vi "display_michelle_PKT_visjitter_stopadded_RandCont_PsuedoCO_TSLogFC2_lightdetection.vi"() -> ()   [LabVIEW 2019]
uses:
  <vilib>/Analysis/Matrix/Datatypes/RealMatrix.ctl
  <vilib>/Utility/file.llb/Write Delimited Spreadsheet (DBL).vi
  <vilib>/Analysis/Matrix/NI_Matrix.lvlib
panel:
  out "LastTimeOutTime":dbl
  out "lambda":dbl
  out "maxITI":dbl
  out "minITI":dbl
  out "goEXP":dbl
  out "meanITI":dbl
  out "Lag1":dbl
  out "TSLog":dbl[][](array[numeric])
  out "TSLog2":dbl[][](array[numeric])
  out "Initialtime":dbl
  out "Time Stamp":timestamp format="%<%H:%M:%S%4u>T"
  out "TSLog1":dbl[][](array[numeric])
  out "ArrayTemp3":T1
  out "StimID2":dbl
  out "Contrast":dbl
  out "TimeOutCounter":i32
  out "ElapsedTime_M":dbl
  out "Base_Contrast":dbl
  out "CurrentTrial":u32=1
  out "Jitter":dbl
  out "BaseITI":dbl
  out "VisStimDuration":dbl
  in  "Stop":bool
  out "Num trials":u32=204
  out "ISI Time":dbl
  out "Stim TS":dbl
  out "Output":dbl[][](array[numeric])
  out "Output frame":T1
  out "Array temp1":T1
  out "Elapsed Time":dbl
  out "Display":bool=TRUE
  out "Trial":u32=1
  out "reward":dbl[](array[numeric])
  out "stim_id":dbl[](array[numeric])
  out "stim_loaded":dbl
  out "Timings":dbl[](array[numeric])
  out "Stimuli Loaded?":bool
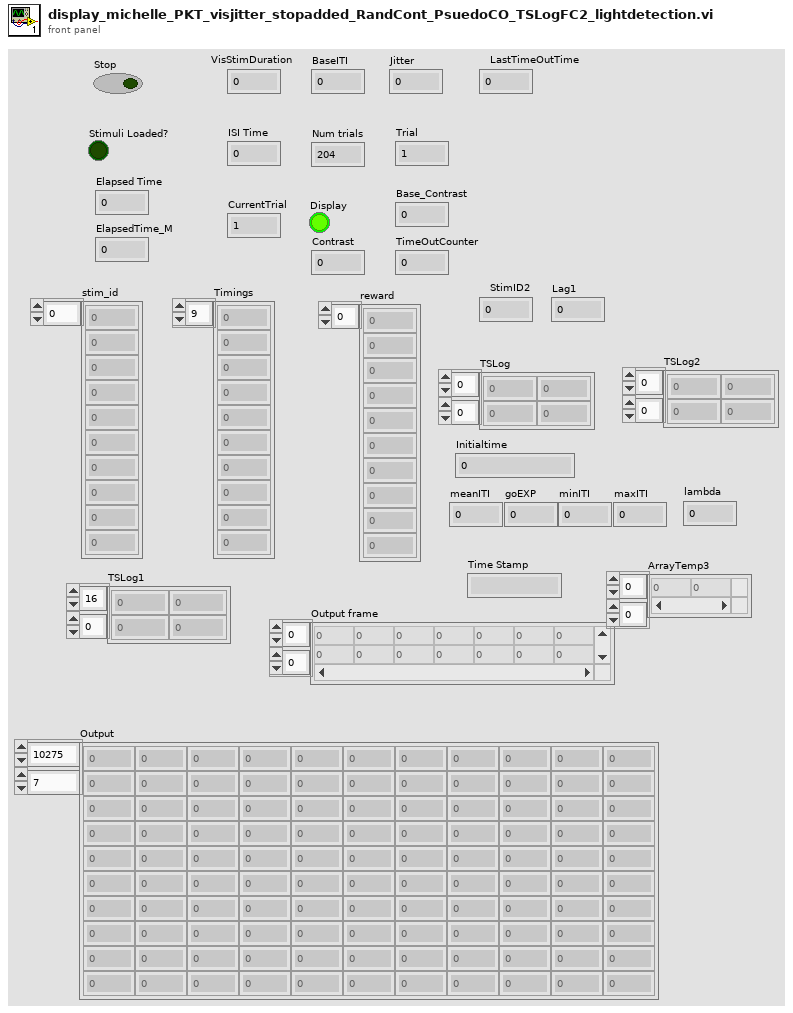
[diagram p1: front panel]
types:
  T1 = typedef "NI_Matrix.lvlib/RealMatrix.ctl" = dbl[][]
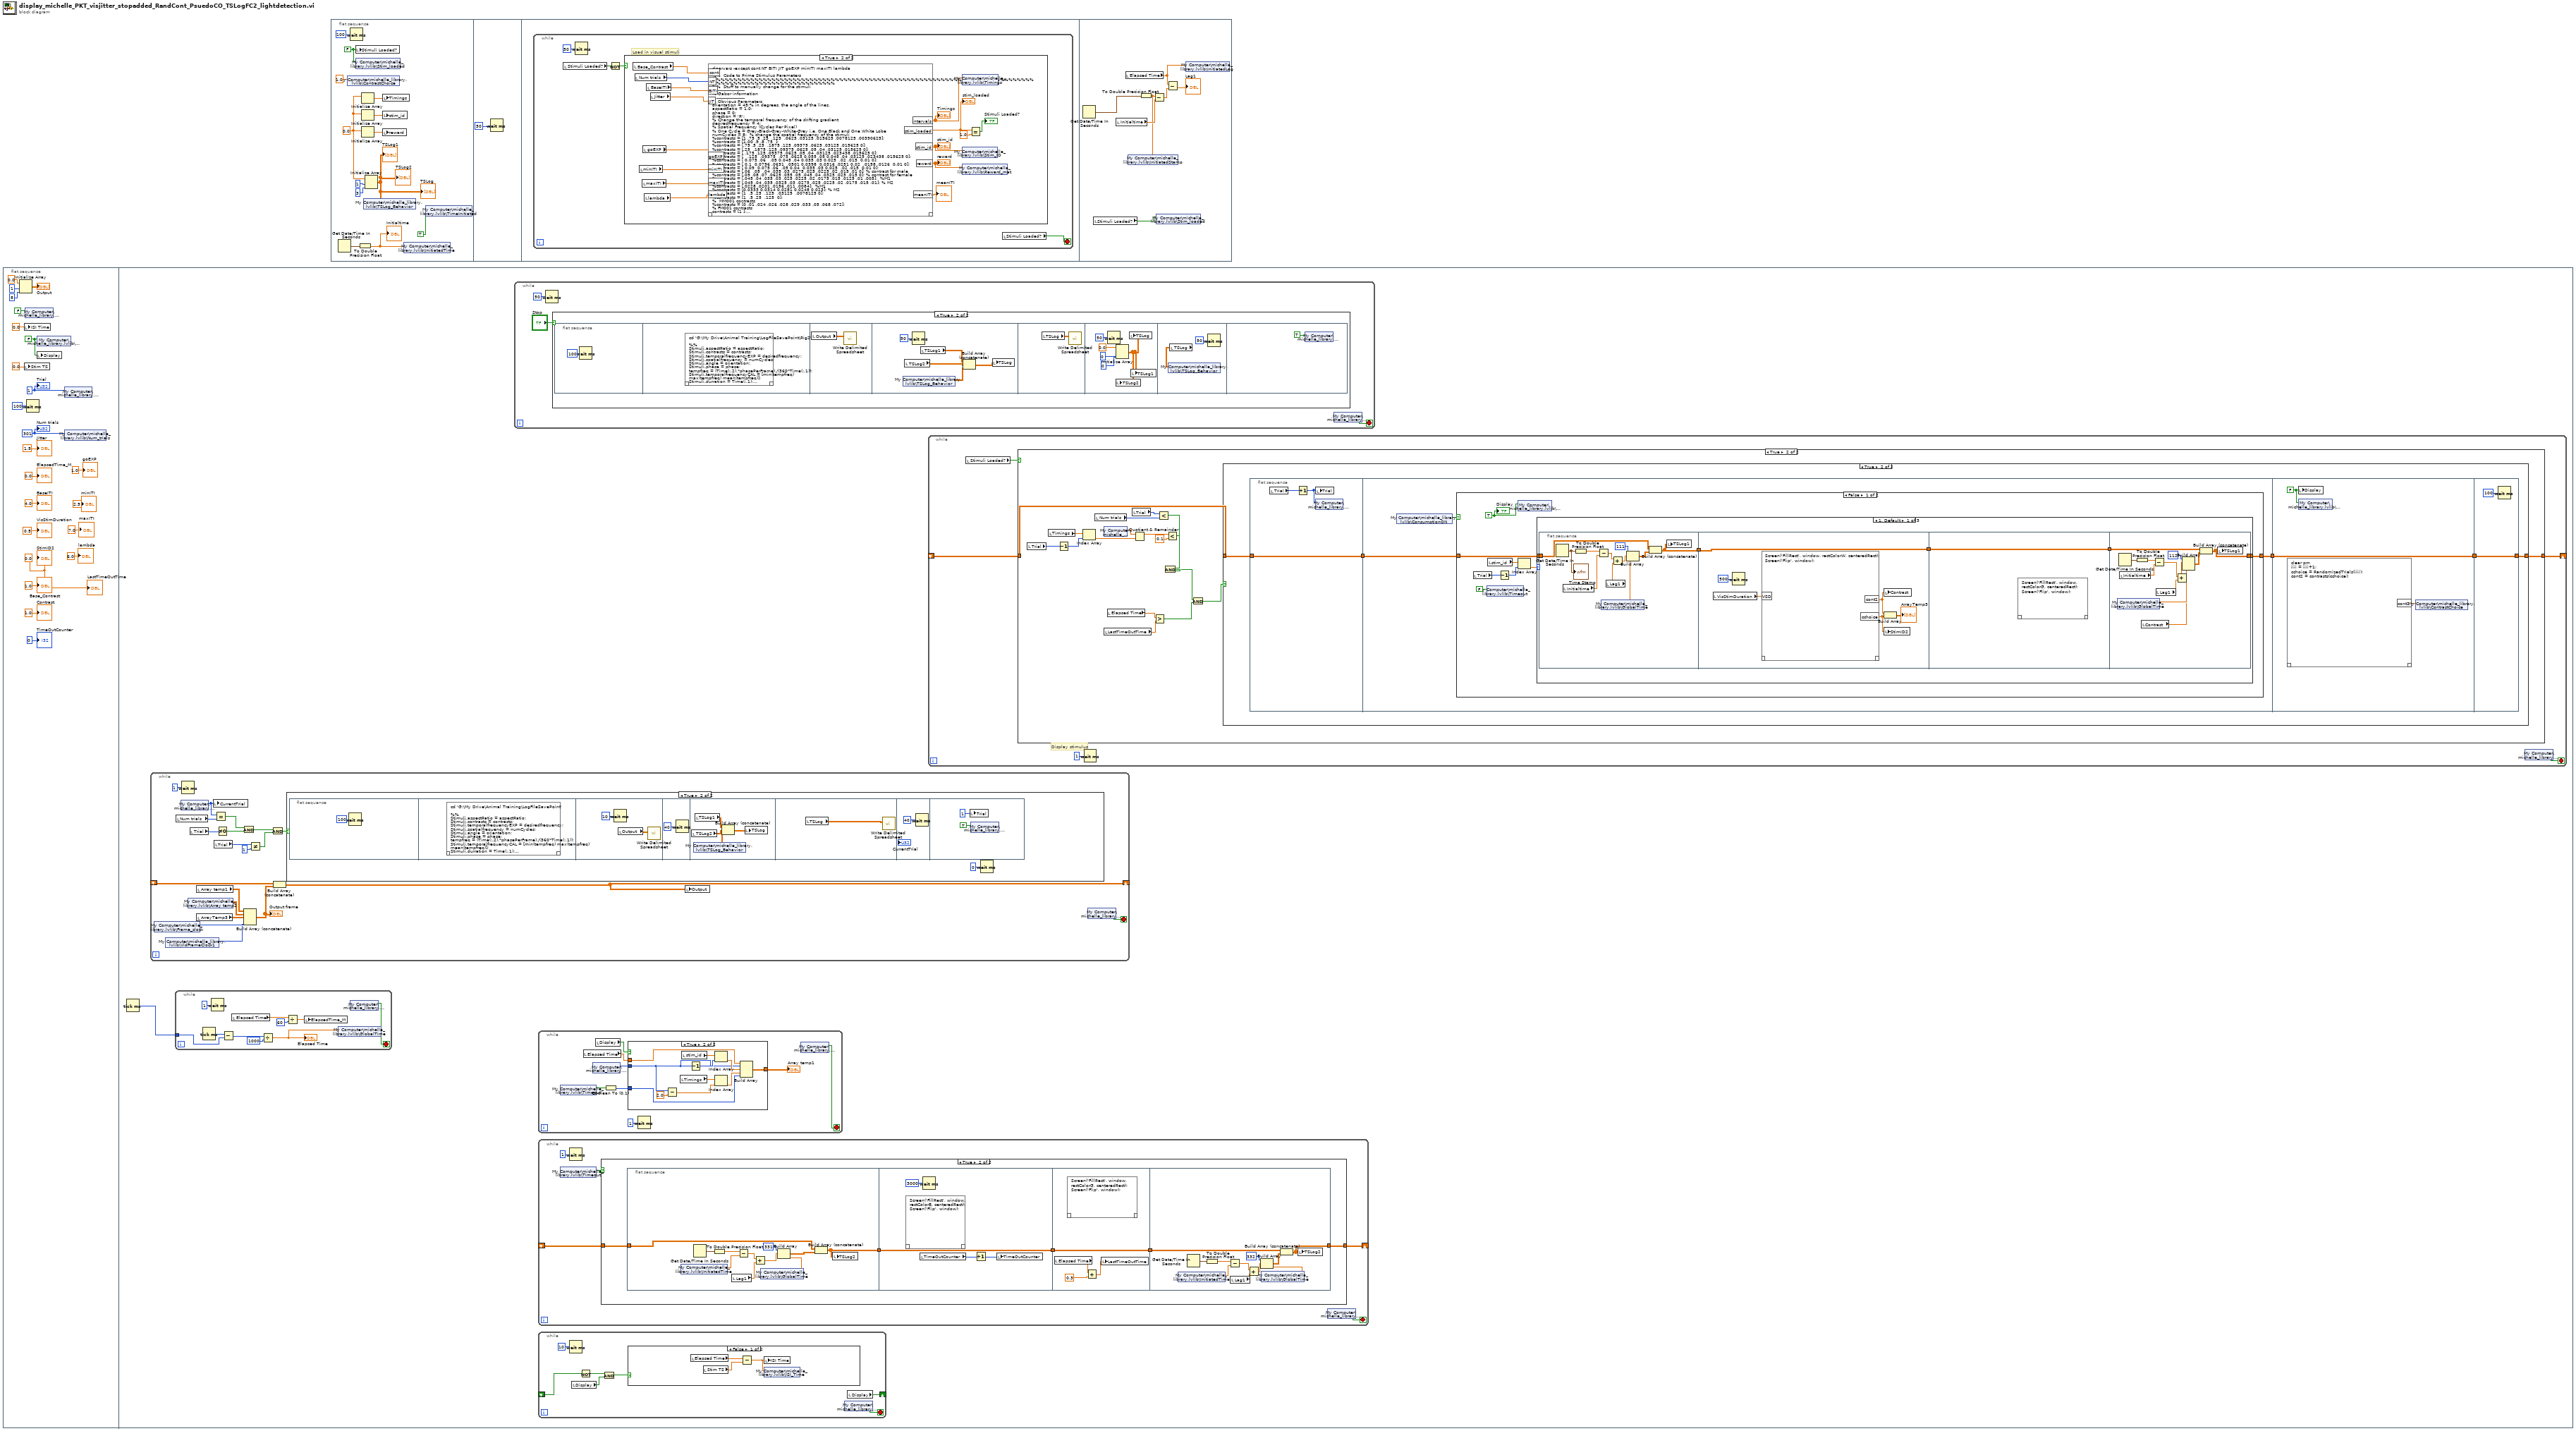
[diagram p0: block diagram]
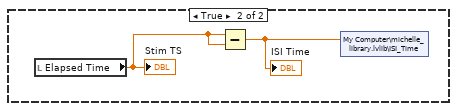
[diagram p5: hidden frame]
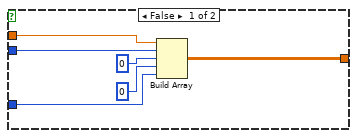
[diagram p6: hidden frame]
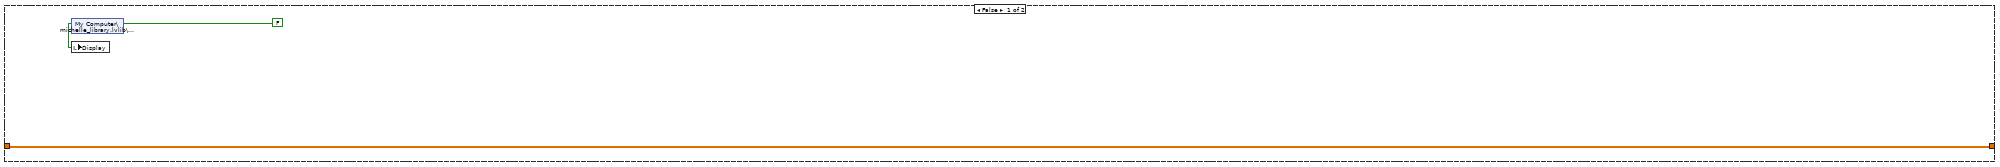
[diagram p9: hidden frame]
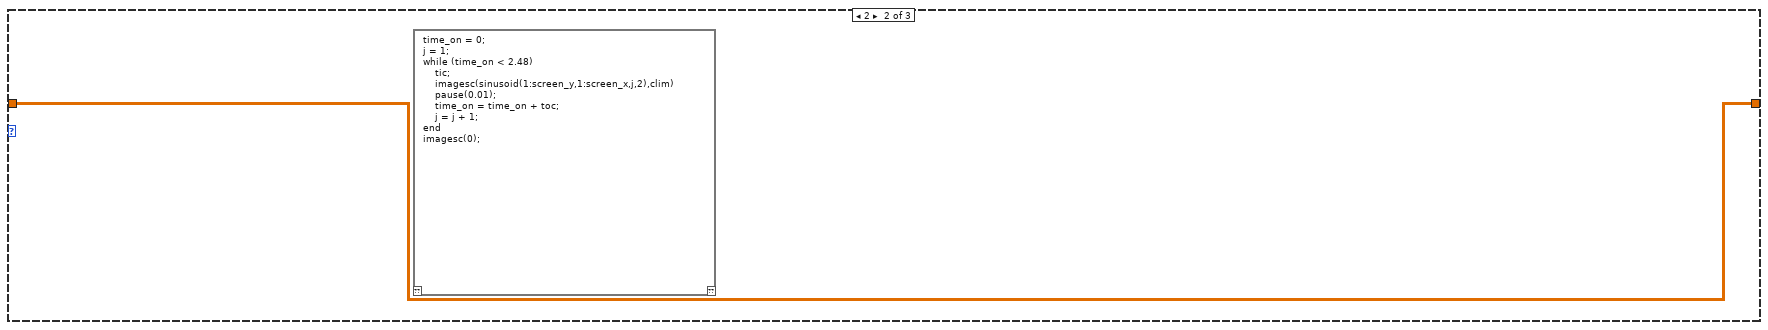
[diagram p10: hidden frame]
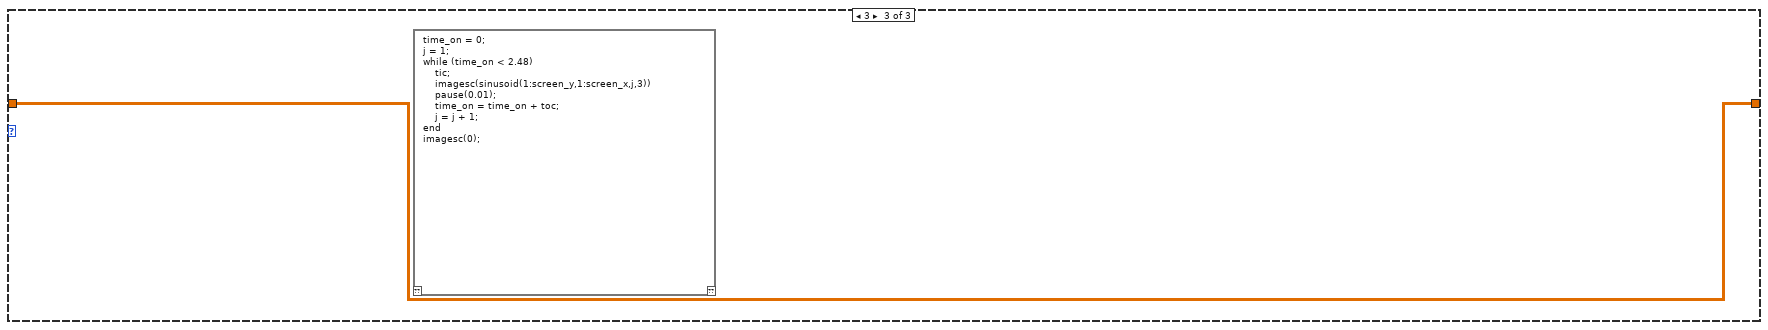
[diagram p11: hidden frame]
diagram:
  n1 = flat-sequence {
    frame #0 {
      w1 = 0.0
      w15 = u32 301
      w21 = FALSE ("Display")
      w23 = u32 1 ("Trial")
      n2 = Initialize Array(0.0 ("element"), 1 ("dimension size"), 8 ("dimension size")) -> (→"Output":dbl[][])
      n3 = local write "ISI Time"(0.0 ("ISI Time")) -> ()
      n4 = local write "Stim TS"(0.0 ("Stim TS")) -> ()
      n5 = shared-variable "My Computer\\michelle_library.lvlib\\Stop"(FALSE ("Stop")) -> ()  [unwired: 1 in, 1 out]
      n6 = Wait (ms)(milliseconds to wait=u32 100) -> ()  [unwired: 1 out]
      n7 = shared-variable "My Computer\\michelle_library.lvlib\\Display"(w21) -> ()  [unwired: 1 in, 1 out]
      n8 = local write "Display"(w21) -> ()
      n9 = shared-variable "My Computer\\michelle_library.lvlib\\Trial"(w23) -> ()  [unwired: 1 in, 1 out]
      n10 = shared-variable "My Computer\\michelle_library.lvlib\\Num_trials"(w15) -> ()  [unwired: 1 in, 1 out]
      "Trial" <- w23
      "Num trials" <- w15
      "VisStimDuration" <- 0.5
      "BaseITI" <- 4.0
      "Jitter" <- 1.5
      "Base_Contrast" <- 1.0
      "ElapsedTime_M" <- 0.0
      "TimeOutCounter" <- 0
      "Contrast" <- 1.0
      "StimID2" <- w1
      "goEXP" <- 1.0
      "minITI" <- 2.5
      "maxITI" <- 7.0
      "lambda" <- 6.0
      "LastTimeOutTime" <- w1
    }
    frame #1 {
      n11 = Tick Count (ms)() -> (millisecond timer value=w24:u32)
      n12 = while {
        shift-right: [w148] -> _
        shift-left: _ -> [w149]
        stop <- w151 stop-if-true
        n13 = shared-variable "My Computer\\michelle_library.lvlib\\Frame_clock"() -> (w133:u32)  [unwired: 1 in, 1 out]
        n14 = shared-variable "My Computer\\michelle_library.lvlib\\VidFrameClock1"() -> (w132:u32)  [unwired: 1 in, 1 out]
        n15 = local read "Num trials"() -> (w144:u32)
        n16 = shared-variable "My Computer\\michelle_library.lvlib\\Trial"() -> (w135:u32)  [unwired: 1 in, 1 out]
        n17 = Wait (ms)(milliseconds to wait=u32 1) -> ()  [unwired: 1 out]
        n18 = shared-variable "My Computer\\michelle_library.lvlib\\Array temp2"() -> (w146:dbl[][])  [unwired: 1 in, 1 out]
        n19 = local read "Trial"() -> (w142:u32)
        n20 = local read "Array temp1"() -> (w147:T1)
        n21 = local read "ArrayTemp3"() -> (w134:T1)
        n22 = local write "CurrentTrial"(w135) -> ()
        n23 = local read "Trial"() -> (w141:u32)
        n24 = Equal?(x=w135, y=w144) -> (x = y?=w143:bool)
        n25 = Not Equal To 0?(x=w142) -> (x != 0?=w138:bool)
        n26 = And(x=w143, y=w138) -> (x .and. y?=w136:bool)
        n27 = Build Array (concatenate)(w147, w146, w134, w133, w132) -> (w145:T1)
        "Output frame" <- w145
        n28 = Not Equal?(x=w141, y=1) -> (x != y?=w140:bool)
        n29 = And(x=w136, y=w140) -> (x .and. y?=w137:bool)
        n30 = Build Array (concatenate) ("Build Matrix")(w149, w145) -> (w148:T1)
        n31 = case shown="True" w137 {
          frame False {
          }
          frame True {
            n32 = flat-sequence {
              frame #0 {
                n33 = Wait (ms)(milliseconds to wait=100) -> ()  [unwired: 1 out]
              }
              frame #1 {
                n34 = script code="cd 'G:\\My Drive\\Animal Training\\LogFileSavePoint'\n\n%%\nStimuli.aspectRatio = aspectRatio;\nStimuli.contrasts = contrasts;\nStimuli.temporalfrequencyEXP = desiredfrequency;\nStimuli.spatialfrequency = numCycles;\nStimuli.angle = orientation;\nStimuli.phase = phase;\ntempfreq = (Time(:,2).*phasePerFrame)./(360*Time(:,1)); \nStimuli.temporalfrequencyCAL = [min(tempfreq) max(tempfreq) mean(tempfreq)];\nStimuli.durration = Time(:,1);\nStimuli.frames = Time(:,2);\nStimuli.contrast = Time(:,3);\nStimuli.intervals = intervals;\nif goEXP == 0\n     int.type = 'jitter';\n     int.baseITI = BITI;\n     int.jitter = JIT;\nelseif goEXP == 1\n     int.type = 'exponential';\n     int.minITI = minITI;\n     int.maxITI = maxITI;\n     int.lambda = lambda;\nend\nStimuli.IntervalData = int;\n\n\nWindow.Xpixels = screenXpixels;\nWindow.Ypixels = screenYpixels;\nWindow.Xcenter = xCenter;\nWindow.Ycenter = yCenter;\nWindow.ifi = ifi;\nWindow.screen = screenNumber;\n\n%%\n[logname] = generatelogname();\n\nsave(logname,'Stimuli','Window');"() -> ()  [unwired: 1 in, 1 out]
              }
              frame #2 {
                n35 = Wait (ms)(milliseconds to wait=u32 10) -> ()  [unwired: 1 out]
                n36 = local read "Output"() -> (w155:dbl[][])
                n37 = call-poly <vilib>:"Write Delimited Spreadsheet.vi"("2D data"=w155) -> ()  [unwired: 13 in, 2 out]
              }
              frame #3 {
                n38 = Wait (ms)(milliseconds to wait=u32 40) -> ()  [unwired: 1 out]
              }
              frame #4 {
                n39 = local read "TSLog2"() -> (w160:dbl[][])
                n40 = shared-variable "My Computer\\michelle_library.lvlib\\TSLog_Behavior"() -> (w158:dbl[][])  [unwired: 1 in, 1 out]
                n41 = local read "TSLog1"() -> (w159:dbl[][])
                n42 = Build Array (concatenate) ("Build Matrix")(w159, w160, w158) -> (w157:T1)
                n43 = local write "TSLog"(w157) -> ()
              }
              frame #5 {
                n44 = local read "TSLog"() -> (w161:dbl[][])
                n45 = call-poly <vilib>:"Write Delimited Spreadsheet.vi"("2D data"=w161) -> ()  [unwired: 13 in, 2 out]
              }
              frame #6 {
                n46 = Wait (ms)(milliseconds to wait=u32 40) -> ()  [unwired: 1 out]
              }
              frame #7 {
                n47 = local write "Trial"(1) -> ()
                n48 = shared-variable "My Computer\\michelle_library.lvlib\\Stop"(TRUE) -> ()  [unwired: 1 in, 1 out]
              }
            }
            n49 = Wait (ms)(milliseconds to wait=0) -> ()  [unwired: 1 out]
          }
        }
        n50 = local write "Output"(w148) -> ()
        n51 = shared-variable "My Computer\\michelle_library.lvlib\\Stop"() -> (w151:bool)  [unwired: 1 in, 1 out]
      }
      n52 = while {
        tunnel: w24 -> [w129]
        stop <- w126 stop-if-true
        n53 = Tick Count (ms)() -> (millisecond timer value=w130:u32)
        n54 = Wait (ms)(milliseconds to wait=u32 1) -> ()  [unwired: 1 out]
        n55 = Subtract(x=w130, y=w129) -> (x-y=w127:u32)
        n56 = local read "Elapsed Time"() -> (w124:dbl)
        n57 = Divide(x=w127, y=u32 1000) -> (x/y=w122:dbl)
        "Elapsed Time" <- w122
        n58 = Divide(x=w124, y=60) -> (x/y=w123:dbl)
        n59 = local write "ElapsedTime_M"(w123) -> ()
        n60 = shared-variable "My Computer\\michelle_library.lvlib\\GlobalTime"(w122) -> ()  [unwired: 1 in, 1 out]
        n61 = shared-variable "My Computer\\michelle_library.lvlib\\Stop"() -> (w126:bool)  [unwired: 1 in, 1 out]
      }
      n62 = while {
        stop <- w27 stop-if-true
        n63 = Wait (ms)(milliseconds to wait=50) -> ()  [unwired: 1 out]
        n64 = case shown="True" "Stop" {
          frame False {
          }
          frame True {
            n65 = flat-sequence {
              frame #0 {
                n66 = Wait (ms)(milliseconds to wait=100) -> ()  [unwired: 1 out]
              }
              frame #1 {
                n67 = script code="cd 'G:\\My Drive\\Animal Training\\LogFileSavePoint\\Rig2'\n\n%%\nStimuli.aspectRatio = aspectRatio;\nStimuli.contrasts = contrasts;\nStimuli.temporalfrequencyEXP = desiredfrequency;\nStimuli.spatialfrequency = numCycles;\nStimuli.angle = orientation;\nStimuli.phase = phase;\ntempfreq = (Time(:,2).*phasePerFrame)./(360*Time(:,1)); \nStimuli.temporalfrequencyCAL = [min(tempfreq) max(tempfreq) mean(tempfreq)];\nStimuli.durration = Time(:,1);\nStimuli.frames = Time(:,2);\nStimuli.contrast = Time(:,3);\nStimuli.intervals = intervals;\nif goEXP == 0\n     int.type = 'jitter';\n     int.baseITI = BITI;\n     int.jitter = JIT;\nelseif goEXP == 1\n     int.type = 'exponential';\n     int.minITI = minITI;\n     int.maxITI = maxITI;\n     int.lambda = lambda;\nend\nStimuli.IntervalData = int;\n\n\nWindow.Xpixels = screenXpixels;\nWindow.Ypixels = screenYpixels;\nWindow.Xcenter = xCenter;\nWindow.Ycenter = yCenter;\nWindow.ifi = ifi;\nWindow.screen = screenNumber;\n\n%%\n[logname] = generatelogname();\n\nsave(logname,'Stimuli','Window');"() -> ()  [unwired: 1 in, 1 out]
              }
              frame #2 {
                n68 = local read "Output"() -> (w29:dbl[][])
                n69 = call-poly <vilib>:"Write Delimited Spreadsheet.vi"("2D data"=w29) -> ()  [unwired: 13 in, 2 out]
              }
              frame #3 {
                n70 = shared-variable "My Computer\\michelle_library.lvlib\\TSLog_Behavior"() -> (w30:dbl[][])  [unwired: 1 in, 1 out]
                n71 = local read "TSLog2"() -> (w33:dbl[][])
                n72 = Wait (ms)(milliseconds to wait=50) -> ()  [unwired: 1 out]
                n73 = local read "TSLog1"() -> (w32:dbl[][])
                n74 = Build Array (concatenate) ("Build Matrix")(w32, w33, w30) -> (w31:T1)
                n75 = local write "TSLog"(w31) -> ()
              }
              frame #4 {
                n76 = local read "TSLog"() -> (w35:dbl[][])
                n77 = call-poly <vilib>:"Write Delimited Spreadsheet.vi"("2D data"=w35) -> ()  [unwired: 13 in, 2 out]
              }
              frame #5 {
                n78 = Wait (ms)(milliseconds to wait=50) -> ()  [unwired: 1 out]
                n79 = Initialize Array(0.0, 0, 0) -> (w37:dbl[][])
                n80 = local write "TSLog2"(w37) -> ()
                n81 = local write "TSLog"(w37) -> ()
                n82 = local write "TSLog1"(w37) -> ()
              }
              frame #6 {
                n83 = local read "TSLog"() -> (w42:dbl[][])
                n84 = shared-variable "My Computer\\michelle_library.lvlib\\TSLog_Behavior"(w42) -> ()  [unwired: 1 in, 1 out]
                n85 = Wait (ms)(milliseconds to wait=50) -> ()  [unwired: 1 out]
              }
              frame #7 {
                n86 = shared-variable "My Computer\\michelle_library.lvlib\\Stop"(TRUE) -> ()  [unwired: 1 in, 1 out]
              }
            }
          }
        }
        n87 = shared-variable "My Computer\\michelle_library.lvlib\\Stop"() -> (w27:bool)  [unwired: 1 in, 1 out]
      }
      n88 = while {
        stop <- w99 stop-if-true
        n89 = shared-variable "My Computer\\michelle_library.lvlib\\Timeout"() -> (w97:bool)  [unwired: 1 in, 1 out]
        n90 = local read "Elapsed Time"() -> (w103:dbl)
        n91 = shared-variable "My Computer\\michelle_library.lvlib\\Trial"() -> (w101:u32)  [unwired: 1 in, 1 out]
        n92 = local read "Display"() -> (w100:bool)
        n93 = Boolean To (0,1)(Boolean=w97) -> (0, 1=w98:i16)
        n94 = case shown="True" w100 {
          tunnel: w101 -> [w109 w112]
          tunnel: w103 -> [w110 w119]
          tunnel: [w108 w120] -> w102
          tunnel: w98 -> [w105 w114]
          frame False {
            n95 = Build Array(w110, w109, u32 0 ("milliseconds to wait"), 0, w105) -> (w108:T1)
          }
          frame True {
            n96 = Subtract(x=w112, y=2.0) -> (x-y=w111:dbl)
            n97 = local read "Timings"() -> (w117:dbl[])
            n98 = local read "stim_id"() -> (w121:dbl[])
            n99 = Decrement(x=w112) -> (x-1=w116:u32)
            n100 = Index Array(array=w121, index=w116) -> (element=w118:dbl)
            n101 = Index Array(array=w117, index=w111) -> (element=w115:dbl)
            n102 = Build Array(w119, w112, w118, w115, w114) -> (w120:T1)
          }
        }
        "Array temp1" <- w102
        n103 = Wait (ms)(milliseconds to wait=u32 1) -> ()  [unwired: 1 out]
        n104 = shared-variable "My Computer\\michelle_library.lvlib\\Stop"() -> (w99:bool)  [unwired: 1 in, 1 out]
      }
      n105 = while {
        shift-right: [w44] -> _
        shift-left: _ -> [w45]
        stop <- w48 stop-if-true
        n106 = shared-variable "My Computer\\michelle_library.lvlib\\Timeout"() -> (w46:bool)  [unwired: 1 in, 1 out]
        n107 = Wait (ms)(milliseconds to wait=u32 1) -> ()  [unwired: 1 out]
        n108 = case shown="True" w46 {
          tunnel: w45 -> [w49 w54]
          tunnel: [w49 w53] -> w44
          frame False {
          }
          frame True {
            n109 = flat-sequence {
              tunnel: w54 -> [w60]
              tunnel: [w59] -> w51
              tunnel: [w66] -> w52
              tunnel: w51 -> [w66]
              tunnel: w52 -> [w73]
              tunnel: [w73] -> w50
              tunnel: [w78] -> w53
              tunnel: w50 -> [w79]
              frame #0 {
                n110 = shared-variable "My Computer\\michelle_library.lvlib\\InitiatedTime"() -> (w63:dbl)  [unwired: 1 in, 1 out]
                n111 = Get Date/Time In Seconds() -> (seconds since 1Jan1904=w65:timestamp)
                n112 = To Double Precision Float(number=w65) -> (double precision float=w64:dbl)
                n113 = local read "Lag1"() -> (w56:dbl)
                n114 = Subtract(x=w64, y=w63) -> (x-y=w57:dbl)
                n115 = Add(x=w57, y=w56) -> (x+y=w58:dbl)
                n116 = shared-variable "My Computer\\michelle_library.lvlib\\GlobalTime"() -> (w55:dbl)  [unwired: 1 in, 1 out]
                n117 = Build Array(331, w58, w55) -> (w62:T1)
                n118 = Build Array (concatenate) ("Build Matrix")(w60, w62) -> (w59:T1)
                n119 = local write "TSLog2"(w59) -> ()
              }
              frame #1 {
                n120 = script code="Screen('FillRect', window, rectColorB, centeredRect);\nScreen('Flip', window);"() -> ()  [unwired: 1 in, 1 out]
                n121 = local read "TimeOutCounter"() -> (w68:i32)
                n122 = Wait (ms)(milliseconds to wait=u32 3000) -> ()  [unwired: 1 out]
                n123 = Increment(x=w68) -> (x+1=w67:i32)
                n124 = local write "TimeOutCounter"(w67) -> ()
              }
              frame #2 {
                n125 = local read "Elapsed Time"() -> (w71:dbl)
                n126 = script code="Screen('FillRect', window, rectColorG, centeredRect);\nScreen('Flip', window);"() -> ()  [unwired: 1 in, 1 out]
                n127 = Add(x=w71, y=0.3) -> (x+y=w72:dbl)
                n128 = local write "LastTimeOutTime"(w72) -> ()
              }
              frame #3 {
                n129 = shared-variable "My Computer\\michelle_library.lvlib\\InitiatedTime"() -> (w84:dbl)  [unwired: 1 in, 1 out]
                n130 = Get Date/Time In Seconds() -> (seconds since 1Jan1904=w82:timestamp)
                n131 = To Double Precision Float(number=w82) -> (double precision float=w83:dbl)
                n132 = Subtract(x=w83, y=w84) -> (x-y=w76:dbl)
                n133 = local read "Lag1"() -> (w75:dbl)
                n134 = Add(x=w76, y=w75) -> (x+y=w77:dbl)
                n135 = shared-variable "My Computer\\michelle_library.lvlib\\GlobalTime"() -> (w74:dbl)  [unwired: 1 in, 1 out]
                n136 = Build Array(332, w77, w74) -> (w80:T1)
                n137 = Build Array (concatenate) ("Build Matrix")(w79, w80) -> (w78:T1)
                n138 = local write "TSLog2"(w78) -> ()
              }
            }
          }
        }
        n139 = shared-variable "My Computer\\michelle_library.lvlib\\Stop"() -> (w48:bool)  [unwired: 1 in, 1 out]
      }
      n140 = while {
        shift-right: [w89] -> _
        shift-left: _ -> [w88]
        stop <- w91 stop-if-true
        n141 = Wait (ms)(milliseconds to wait=u32 10) -> ()  [unwired: 1 out]
        n142 = local read "Display"() -> (w86:bool)
        n143 = Not(x=w88) -> (.not. x?=w87:bool)
        n144 = And(x=w87, y=w86) -> (x .and. y?=w85:bool)
        n145 = case shown="False" w85 {
          frame False {
            n146 = local read "Elapsed Time"() -> (w92:dbl)
            n147 = local read "Stim TS"() -> (w94:dbl)
            n148 = Subtract(x=w92, y=w94) -> (x-y=w93:dbl)
            n149 = local write "ISI Time"(w93) -> ()
            n150 = shared-variable "My Computer\\michelle_library.lvlib\\ISI_Time"(w93) -> ()  [unwired: 1 in, 1 out]
          }
          frame True {
            n151 = local read "Elapsed Time"() -> (w95:dbl)
            "Stim TS" <- w95
            n152 = Subtract(x=w95, y=w95) -> (x-y=w96:dbl)
            "ISI Time" <- w96
            n153 = shared-variable "My Computer\\michelle_library.lvlib\\ISI_Time"(w96) -> ()  [unwired: 1 in, 1 out]
          }
        }
        n154 = shared-variable "My Computer\\michelle_library.lvlib\\Stop"() -> (w91:bool)  [unwired: 1 in, 1 out]
        n155 = local read "Display"() -> (w89:bool)
      }
      n156 = while {
        shift-right: [w165] -> _
        shift-left: _ -> [w166]
        stop <- w168 stop-if-true
        # "Display stimulus"
        n157 = local read "Stimuli Loaded?"() -> (w167:bool)
        n158 = case shown="True" w167 {
          tunnel: w166 -> [w170 w177]
          tunnel: [w170 w176] -> w165
          frame False {
          }
          frame True {
            n159 = local read "Trial"() -> (w178:u32)
            n160 = local read "Timings"() -> (w186:dbl[])
            n161 = Decrement(x=w178) -> (x-1=w179:u32)
            n162 = Index Array(array=w186, index=w179) -> (element=w185:dbl)
            n163 = local read "Num trials"() -> (w181:u32)
            n164 = shared-variable "My Computer\\michelle_library.lvlib\\ISI"() -> (w180:dbl)  [unwired: 1 in, 1 out]
            n165 = local read "LastTimeOutTime"() -> (w171:dbl)
            n166 = local read "Elapsed Time"() -> (w173:dbl)
            n167 = local read "Trial"() -> (w184:u32)
            n168 = Quotient & Remainder(x=w180, y=w185) -> (x-y*floor(x/y)=w188:dbl)  [unwired: 1 out]
            n169 = Greater?(x=w173, y=w171) -> (0:w172:bool)
            n170 = Less?(x=w184, y=w181) -> (x < y?=w183:bool)
            n171 = Less?(x=w188, y=0.1) -> (x < y?=w182:bool)
            n172 = And(x=w183, y=w182) -> (x .and. y?=w175:bool)
            n173 = And(x=w175, y=w172) -> (x .and. y?=w174:bool)
            n174 = case shown="True" w174 {
              tunnel: w177 -> [w189 w194]
              tunnel: [w189 w193] -> w176
              frame False {
                w190 = FALSE ("Display")
                n175 = shared-variable "My Computer\\michelle_library.lvlib\\Display"(w190) -> ()  [unwired: 1 in, 1 out]
                n176 = local write "Display"(w190) -> ()
              }
              frame True {
                n177 = flat-sequence {
                  tunnel: [w196] -> w195
                  tunnel: w194 -> [w196]
                  tunnel: w195 -> [w200]
                  tunnel: [w199] -> w191
                  tunnel: [w248] -> w192
                  tunnel: w191 -> [w248]
                  tunnel: [w251] -> w193
                  tunnel: w192 -> [w251]
                  frame #0 {
                    n178 = local read "Trial"() -> (w198:u32)
                    n179 = Increment(x=w198) -> (x+1=w197:u32)
                    n180 = local write "Trial"(w197) -> ()
                    n181 = shared-variable "My Computer\\michelle_library.lvlib\\Trial"(w197) -> ()  [unwired: 1 in, 1 out]
                  }
                  frame #1 {
                    n182 = shared-variable "My Computer\\michelle_library.lvlib\\ConsumptionON"() -> (w201:bool)  [unwired: 1 in, 1 out]
                    n183 = case shown="False" w201 {
                      tunnel: w200 -> [w203 w247]
                      tunnel: [w202 w247] -> w199
                      frame False {
                        w204 = TRUE ("Boolean")
                        n184 = local read "Trial"() -> (w207:u32)
                        n185 = shared-variable "My Computer\\michelle_library.lvlib\\Timeout"(FALSE) -> ()  [unwired: 1 in, 1 out]
                        n186 = local read "stim_id"() -> (w209:dbl[])
                        n187 = Decrement(x=w207) -> (x-1=w206:u32)
                        n188 = shared-variable "My Computer\\michelle_library.lvlib\\Display"(w204) -> ()  [unwired: 1 in, 1 out]
                        n189 = Index Array(array=w209, index=w206) -> (element=w208:dbl)
                        n190 = case shown="1, Default" w208 {
                          tunnel: w203 -> [w214 w245 w246]
                          tunnel: [w213 w245 w246] -> w202
                          frame 1, Default {
                            n191 = flat-sequence {
                              tunnel: w214 -> [w224]
                              tunnel: [w223] -> w212
                              tunnel: w212 -> [w227]
                              tunnel: [w227] -> w211
                              tunnel: w211 -> [w232]
                              tunnel: [w232] -> w210
                              tunnel: [w243] -> w213
                              tunnel: w210 -> [w242]
                              frame #0 {
                                n192 = Get Date/Time In Seconds() -> (seconds since 1Jan1904=w221:timestamp)
                                "Time Stamp" <- w221
                                n193 = local read "Initialtime"() -> (w219:dbl)
                                n194 = To Double Precision Float(number=w221) -> (double precision float=w220:dbl)
                                n195 = Subtract(x=w220, y=w219) -> (x-y=w217:dbl)
                                n196 = shared-variable "My Computer\\michelle_library.lvlib\\GlobalTime"() -> (w215:dbl)  [unwired: 1 in, 1 out]
                                n197 = local read "Lag1"() -> (w218:dbl)
                                n198 = Add(x=w217, y=w218) -> (x+y=w216:dbl)
                                n199 = Build Array(111, w216, w215) -> (w222:T1)
                                n200 = Build Array (concatenate) ("Build Matrix")(w224, w222) -> (w223:T1)
                                n201 = local write "TSLog1"(w223) -> ()
                              }
                              frame #1 {
                                n202 = local read "VisStimDuration"() -> (w229:dbl)
                                n203 = Wait (ms)(milliseconds to wait=u32 500) -> ()  [unwired: 1 out]
                                n204 = script code="Screen('FillRect', window, rectColorW, centeredRect);\nScreen('Flip', window);"("VSD"=w229) -> ("cont2"=w231:dbl, "cchoice"=w230:dbl)  [unwired: 1 in, 1 out]
                                n205 = local write "Contrast"(w231) -> ()
                                n206 = Build Array(w231, w230) -> (→"ArrayTemp3":T1)
                                n207 = local write "StimID2"(w230) -> ()
                              }
                              frame #2 {
                                n208 = script code="Screen('FillRect', window, rectColorG, centeredRect);\nScreen('Flip', window);"() -> ()  [unwired: 1 in, 1 out]
                              }
                              frame #3 {
                                n209 = shared-variable "My Computer\\michelle_library.lvlib\\GlobalTime"() -> (w234:dbl)  [unwired: 1 in, 1 out]
                                n210 = Get Date/Time In Seconds() -> (seconds since 1Jan1904=w240:timestamp)
                                n211 = local read "Initialtime"() -> (w239:dbl)
                                n212 = To Double Precision Float(number=w240) -> (double precision float=w238:dbl)
                                n213 = local read "Contrast"() -> (w233:dbl)
                                n214 = Subtract(x=w238, y=w239) -> (x-y=w237:dbl)
                                n215 = local read "Lag1"() -> (w235:dbl)
                                n216 = Add(x=w237, y=w235) -> (x+y=w236:dbl)
                                n217 = Build Array(112, w236, w234, w233) -> (w244:T1)
                                n218 = Build Array (concatenate) ("Build Matrix")(w242, w244) -> (w243:T1)
                                n219 = local write "TSLog1"(w243) -> ()
                              }
                            }
                          }
                          frame 2 {
                            n220 = script code="time_on = 0;\nj = 1;\nwhile (time_on < 2.48)\n    tic;\n    imagesc(sinusoid(1:screen_y,1:screen_x,j,2),clim)\n    pause(0.01);\n    time_on = time_on + toc;\n    j = j + 1;\nend\nimagesc(0);"() -> ()  [unwired: 1 in, 1 out]
                          }
                          frame 3 {
                            n221 = script code="time_on = 0;\nj = 1;\nwhile (time_on < 2.48)\n    tic;\n    imagesc(sinusoid(1:screen_y,1:screen_x,j,3))\n    pause(0.01);\n    time_on = time_on + toc;\n    j = j + 1;\nend\nimagesc(0);"() -> ()  [unwired: 1 in, 1 out]
                          }
                        }
                        "Display" <- w204
                      }
                      frame True {
                      }
                    }
                  }
                  frame #2 {
                    w250 = FALSE ("Display")
                    n222 = script code="clear pm\niiii = iiii+1;\ncchoice = RandomizedTrials(iiii);\ncont2 = contrasts(cchoice);"() -> ("cont2"=w249:dbl)  [unwired: 1 in, 1 out]
                    n223 = local write "Display"(w250) -> ()
                    n224 = shared-variable "My Computer\\michelle_library.lvlib\\Display"(w250) -> ()  [unwired: 1 in, 1 out]
                    n225 = shared-variable "My Computer\\michelle_library.lvlib\\ContrastChoice"(w249) -> ()  [unwired: 1 in, 1 out]
                  }
                  frame #3 {
                    n226 = Wait (ms)(milliseconds to wait=u32 100) -> ()  [unwired: 1 out]
                  }
                }
              }
            }
          }
        }
        n227 = Wait (ms)(milliseconds to wait=u32 1) -> ()  [unwired: 1 out]
        n228 = shared-variable "My Computer\\michelle_library.lvlib\\Stop"() -> (w168:bool)  [unwired: 1 in, 1 out]
      }
    }
  }
  n229 = flat-sequence {
    frame #0 {
      w259 = 0.0 ("element")
      w261 = FALSE ("Stimuli Loaded?")
      n230 = Get Date/Time In Seconds() -> (seconds since 1Jan1904=w256:timestamp)
      n231 = shared-variable "My Computer\\michelle_library.lvlib\\ContrastChoice"(1.0) -> ()  [unwired: 1 in, 1 out]
      n232 = Wait (ms)(milliseconds to wait=u32 100) -> ()  [unwired: 1 out]
      n233 = local write "Stimuli Loaded?"(w261) -> ()
      n234 = shared-variable "My Computer\\michelle_library.lvlib\\Stim_loaded"(w261) -> ()  [unwired: 1 in, 1 out]
      n235 = To Double Precision Float(number=w256) -> (double precision float=w255:dbl)
      "Initialtime" <- w255
      n236 = Initialize Array(w259) -> (w264:dbl[])  [unwired: 1 in]
      n237 = Initialize Array(w259) -> (w263:dbl[])  [unwired: 1 in]
      n238 = Initialize Array(w259) -> (w262:dbl[])  [unwired: 1 in]
      n239 = Initialize Array(w259, 1, 3) -> (w253:dbl[][])
      "TSLog1" <- w253
      "TSLog2" <- w253
      "TSLog" <- w253
      n240 = shared-variable "My Computer\\michelle_library.lvlib\\TSLog_Behavior"(w253) -> ()  [unwired: 1 in, 1 out]
      n241 = local write "Timings"(w264) -> ()
      n242 = local write "stim_id"(w263) -> ()
      n243 = local write "reward"(w262) -> ()
      n244 = shared-variable "My Computer\\michelle_library.lvlib\\InitiatedTime"(w255) -> ()  [unwired: 1 in, 1 out]
      n245 = shared-variable "My Computer\\michelle_library.lvlib\\TimeInitiated"(TRUE) -> ()  [unwired: 1 in, 1 out]
    }
    frame #1 {
      n246 = Wait (ms)(milliseconds to wait=u32 50) -> ()  [unwired: 1 out]
    }
    frame #2 {
      n247 = while {
        stop <- w267 stop-if-true
        # "Load in visual stimuli"
        n248 = local read "Stimuli Loaded?"() -> (w269:bool)
        n249 = Wait (ms)(milliseconds to wait=u32 50) -> ()  [unwired: 1 out]
        n250 = Not(x=w269) -> (.not. x?=w268:bool)
        n251 = case shown="True" w268 {
          frame False {
          }
          frame True {
            n252 = local read "Base_Contrast"() -> (w277:dbl)
            n253 = local read "Num trials"() -> (w280:u32)
            n254 = local read "minITI"() -> (w273:dbl)
            n255 = local read "maxITI"() -> (w272:dbl)
            n256 = local read "goEXP"() -> (w274:dbl)
            n257 = local read "lambda"() -> (w271:dbl)
            n258 = local read "BaseITI"() -> (w279:dbl)
            n259 = local read "Jitter"() -> (w278:dbl)
            n260 = script code="clearvars -except cont NT BITI JIT goEXP minITI maxITI lambda\n\n%%  Code to Prime Stimulus Parameters\n%%%%%%%%%%%%%%%%%%%%%%%%%%%%%%%%%%%%%%%%%%%%%%%%%%%%%%%%%%%%%%%%%%%%%%%%%%%%%%%%%%%%%%%%%%%%%%%%%%%%%%%%%\n%%  Stuff to manually change for the stimuli\n%--------------------\n% Gabor information\n%--------------------\n% Obvious Parameters\norientation = 45;% in degrees, the angle of the lines.\naspectRatio = 1.0;\nphase = 0;\ndirection = 'R';\n% Change the temporal frequency of the drifting gradient\ndesiredfrequency = 4;\n% Spatial Frequency (Cycles Per Pixel)\n% One Cycle = Grey-Black-Grey-White-Grey i.e. One Black and One White Lobe\nnumCycles = 8;  % change the spatial frequency of the stimuli\n%contrasts = [1 .75 .5 .25  .125  .0625 .03125 .015625 .0078125 .00390625];\n%contrasts = [1.00 .9 .8 .75  ];\n%contrasts = [.75 .5 .25  .1875 .125 .09375 .0625 .03125 .015625 0];\n%contrasts = [.25  .1875 .125 .09375 .0625 .05 .04 .03125 .015625 0];\n%contrasts = [ .175 .125 .09375 .0625 .05 .04 .03125 .023438 .015625 0];\n%contrasts = [   .125  .09375  .075 .0625 0.055 .05 0.045 .04 .03125 .023438 .015625 0];\n%contrasts = [ 0.075 .06   .05 0.045 .04 0.035 .03 0.025  .02 .015  0.01 0];\n%contrasts = [ 0.1  0.0796 .0631  .0501 0.0398  0.0316 .0251 0.02  .0158 .0126  0.01 0];\n%contrasts = [ 0.09  0.075 .06  .05 0.04  0.035 .03 0.025  .02 .015  0.01 0];\n%contrasts = [.06  .05  .04 .035 .03 .0275 .025 .0225 .02 .015 .01 0]; % contrast for male\n%contrasts = [.09 .08 .07 .0625 .055 .05 .045 .04 .0325 .025 .015 0]; % contrast for female\n%contrasts = [.045 .04 .035 .03 .025 .0225 .02 .0175 .015 .0125 .01 .005];  %M1\n%contrasts = [.045 .04 .035 .0325 .03 .0275 .025 .0225 .02 .0175 .015 .01]; % M2\n%contrasts = [.0228 .0201 .0156 .011 .0084];  %M1\n%contrasts = [0.0333 0.0314 0.0281 0.0248 0.023]; % M2\n%contrasts = [1  .5 .25  .125  .03125  .0078125 0];\n%contrasts = [1  .5 .25  .125  0];\n%  MM001 contrasts\n%contrasts = [0 .01 .024 .026 .028 .029 .033 .05 .068 .072];\n% FM001 contrasts\ncontrasts = [1 ];\n\ngo = 1;\nmaxc = round(numel(contrasts)/2);\n%%  To be run of not using exponential\n%%%%%%%%%%%%%%%%%%%%%%%%%%%%%%%%%%%%%%%%%%%%%%%%%%%%%%%%%%%%%%%%%%%%%%%%%%%%%%%%%%%%%%\n% This code will randomize the order of contrasts being presented\n[RandomizedTrials]=RandomizeTrials_Psuedo_function(contrasts,NT,'n');\n\n% This code will generate inter trial intervals with either random jitter\n% or based on an exponential distribution\nif goEXP < 1\n     jit = JIT;\n     jitter = rand(1,NT);\n     jitter = 2*jit*(jitter- .5);\n     ITIbase = BITI;\n     intervals = [ones(1,NT)*ITIbase];\n     intervals = intervals + jitter;\nelseif goEXP > 0\n     intervals = exponentialITI(1/lambda, minITI, maxITI, NT);\nend\n\n%%  Prep the stimulus presentation software\n%%%%%%%%%%%%%%%%%%%%%%%%%%%%%%%%%%%%%%%%%%%%%%%%%%%%%%%%%%%%%%%%%%%%%%%%%%%\nScreen('Preference', 'SkipSyncTests', 1);\nsca;\nclose all;\n% Setup PTB with some default values\nPsychDefaultSetup(2);\n% Set the screen number to the external secondary monitor if there is one connected\nscreenNumber = max(Screen('Screens'));\n\n% Define black, white and grey\nwhite = WhiteIndex(screenNumber);\nblack = BlackIndex(screenNumber);\ngrey = white / 2;\n\n% Open the screen & define it's dimensions\n[window, windowRect] = PsychImaging('OpenWindow', screenNumber, grey,...\n    [], 32, 2, [], [], kPsychNeedRetinaResolution);\n[screenXpixels, screenYpixels] = Screen('WindowSize', window);\n[xCenter, yCenter] = RectCenter(windowRect);\n\n% Get the vertical refresh rate of the monitor\nifi = Screen('GetFlipInterval', window);\n\n% Set maximum priority level\ntopPriorityLevel = MaxPriority(window);\nPriority(topPriorityLevel);\n\n\n% Build a procedural gabor texture (Note: to get a \"standard\" Gabor patch\n% we set a grey background offset, disable normalisation, and set a\n% pre-contrast multiplier of 0.5).\n% Dimension of the region where will draw the Gabor in pixels\ngaborDimPix = windowRect(3);\n% Sigma of Gaussian  (how much to fade around the edges)\nsigma = gaborDimPix / 0;  % change the 0 value to alter the fading\nphasePerFrame = desiredfrequency*360*ifi;\nfreq = numCycles / gaborDimPix;\n\nbackgroundOffset = [0.5 0.5 0.5 0.0];\ndisableNorm = 1;\npreContrastMultiplier = 0.5;\ngabortex = CreateProceduralGabor(window, gaborDimPix, gaborDimPix, [],...\n    backgroundOffset, disableNorm, preContrastMultiplier);\n\n% Randomise the phase of the Gabors and make a properties matrix.\nfor N = 1:numel(contrasts)\npropertiesMat{1,N} = [phase, freq, sigma, contrasts(N), aspectRatio, 0, 0, 0];\nend\n\niiii = 1;\ncchoice = RandomizedTrials(iiii);\ncont2 = contrasts(cchoice);\npm = propertiesMat{1,1};\ncurtrial = 0;\n\n%%  Build up the rectangles for the pause and hold screen\nbaseRect = [0 0 screenXpixels screenYpixels];\ncenteredRect = CenterRectOnPointd(baseRect, xCenter, yCenter);\nrectColorB = [0 0 0];\nrectColorG = [128 128 128]/255;\nrectColorW = [1 1 1];\n\n%%  Finalize the trial data and orders\nstim_id = [ones(1,NT)*1];\nreward = [ones(1,NT)*1];\nmeanITI = nanmean(intervals);\nrand_idx1 = randperm(NT);\nrand_idx2 = randperm(NT);\nintervals = intervals(rand_idx2);\nstim_id = stim_id(rand_idx2);\nreward = reward(rand_idx2);\n%%  All Done!\n%  indicate that the necessary preloading of data has been completed.\nstim_loaded = 1;" ("Script Node")("NT"=w280, "BITI"=w279, "JIT"=w278, "cont"=w277, "goEXP"=w274, "minITI"=w273, "maxITI"=w272, "lambda"=w271) -> ("stim_loaded"=w285:dbl, "intervals"=w281:dbl[], "stim_id"=w282:dbl[], "reward"=w283:dbl[], "meanITI"=→"meanITI":dbl)  [unwired: 1 in, 1 out]
            "stim_loaded" <- w285
            "Timings" <- w281
            "stim_id" <- w282
            "reward" <- w283
            n261 = shared-variable "My Computer\\michelle_library.lvlib\\Timings"(w281) -> ()  [unwired: 1 in, 1 out]
            n262 = shared-variable "My Computer\\michelle_library.lvlib\\Stim_ID"(w282) -> ()  [unwired: 1 in, 1 out]
            n263 = shared-variable "My Computer\\michelle_library.lvlib\\Reward_mat"(w283) -> ()  [unwired: 1 in, 1 out]
            n264 = Equal?(x=w285, y=1.0) -> (x = y?=→"Stimuli Loaded?":bool)
          }
        }
        n265 = local read "Stimuli Loaded?"() -> (w267:bool)
      }
    }
    frame #3 {
      n266 = Get Date/Time In Seconds() -> (seconds since 1Jan1904=w292:timestamp)
      n267 = local read "Stimuli Loaded?"() -> (w287:bool)
      n268 = local read "Initialtime"() -> (w291:dbl)
      n269 = local read "Elapsed Time"() -> (w286:dbl)
      n270 = To Double Precision Float(number=w292) -> (double precision float=w289:dbl)
      n271 = shared-variable "My Computer\\michelle_library.lvlib\\InitiatedStamp"(w289) -> ()  [unwired: 1 in, 1 out]
      n272 = Subtract(x=w289, y=w291) -> (x-y=w290:dbl)
      n273 = shared-variable "My Computer\\michelle_library.lvlib\\Stim_loaded"(w287) -> ()  [unwired: 1 in, 1 out]
      n274 = Subtract(x=w286, y=w290) -> (x-y=→"Lag1":dbl)
      n275 = shared-variable "My Computer\\michelle_library.lvlib\\InitiatedLag"(w286) -> ()  [unwired: 1 in, 1 out]
    }
  }
